vi "Build_Flow_Task.vi"(5 "minimum value":dbl=-5.0 format="%0.2f", 6 "sample mode":i32(ring)=10178 items=["Finite Samples"=10178, "Continuous Samples"=10123, "Hardware Timed Single Point"=12522], 7 "maximum value":dbl=5.0 format="%0.2f", 8 "error in":errorcluster, 9 "rate":dbl=1000.0 format="%0.2f", 10 "physical channels":tag, 11 "samples per channel":i32=1000) -> (0 "error out":errorcluster, 3 "task out":refnum<k21>)   [LabVIEW 2019]
uses:
  <vilib>/DAQmx/create/channels.llb/DAQmx Create Channel (AI-Voltage-Basic).vi
  <vilib>/DAQmx/configure/timing.llb/DAQmx Timing (Sample Clock).vi
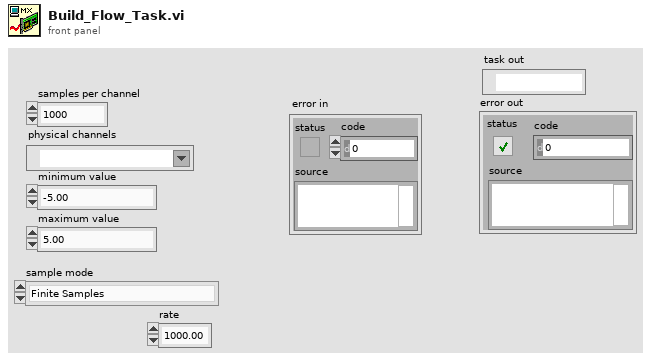
[diagram p1: front panel]
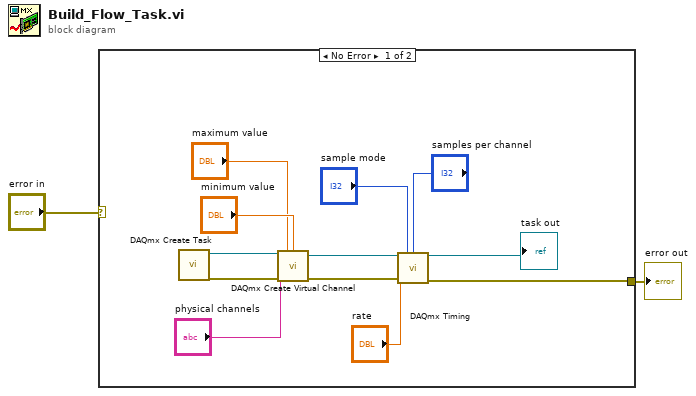
[diagram p0: block diagram]
diagram:
  n1 = case shown="No Error" "error in" {
    selector: "error in" -> [_ w15]
    tunnel: [w8 w15] -> w2
    frame No Error {
      n2 = call <vilib>:"DAQmx Create Task.vi"() -> ("task out"=w14:refnum<k21>, "error out"=w13:errorcluster)  [unwired: 14 in]
      n3 = call-poly <vilib>:"DAQmx Create Virtual Channel.vi"("task in"=w14, "maximum value"="maximum value", "minimum value"="minimum value", "physical channels"="physical channels", "error in"=w13) -> ("task out"=w12:refnum<k21>, "error out"=w11:errorcluster)  [unwired: 9 in]
      n4 = call-poly <vilib>:"DAQmx Timing.vi"("task/channels in"=w12, "sample mode"="sample mode", "samples per channel"="samples per channel", "rate"="rate", "error in"=w11) -> ("task out"=→"task out":refnum<k21>, "error out"=w8:errorcluster)  [unwired: 9 in]
    }
    frame Error {
    }
  }
  "error out" <- w2
